vi "Get Profile Data.vi"(8 "error in (no error)":errorcluster, 10 "Bitfile Path":path, 11 "Profile Data In":T1[](array[typedef])) -> (1 "List of IO interfaces":T2[](array[typedef]), 3 "Profile Data Out":T1[](array[typedef]))   [LabVIEW 2021]
uses:
  <vilib>/myRIO/Common/Instrument Driver Framework/Utilities/typedefs/Hardware Version Enum.ctl
  <vilib>/myRIO/Common/Profile Manager Framework/typedefs/Channel Type Profile.ctl
  <vilib>/myRIO/Common/Instrument Driver Framework/Utilities/typedefs/Channel Types.ctl
  <vilib>/myRIO/Common/Profile Manager Framework/typedefs/Channel Info.ctl
  <vilib>/myRIO/Common/Instrument Driver Framework/Utilities/typedefs/Channel List Array.ctl
  <vilib>/myRIO/Common/Instrument Driver Framework/Utilities/typedefs/Channel List Cluster.ctl
  <vilib>/rvi/Bitfile/niFpgaBitfileReadAction.ctl
panel:
  out "Read Bitfile Time":u32
  in  "Hardware Version":T4=enum."myRIO-1900"
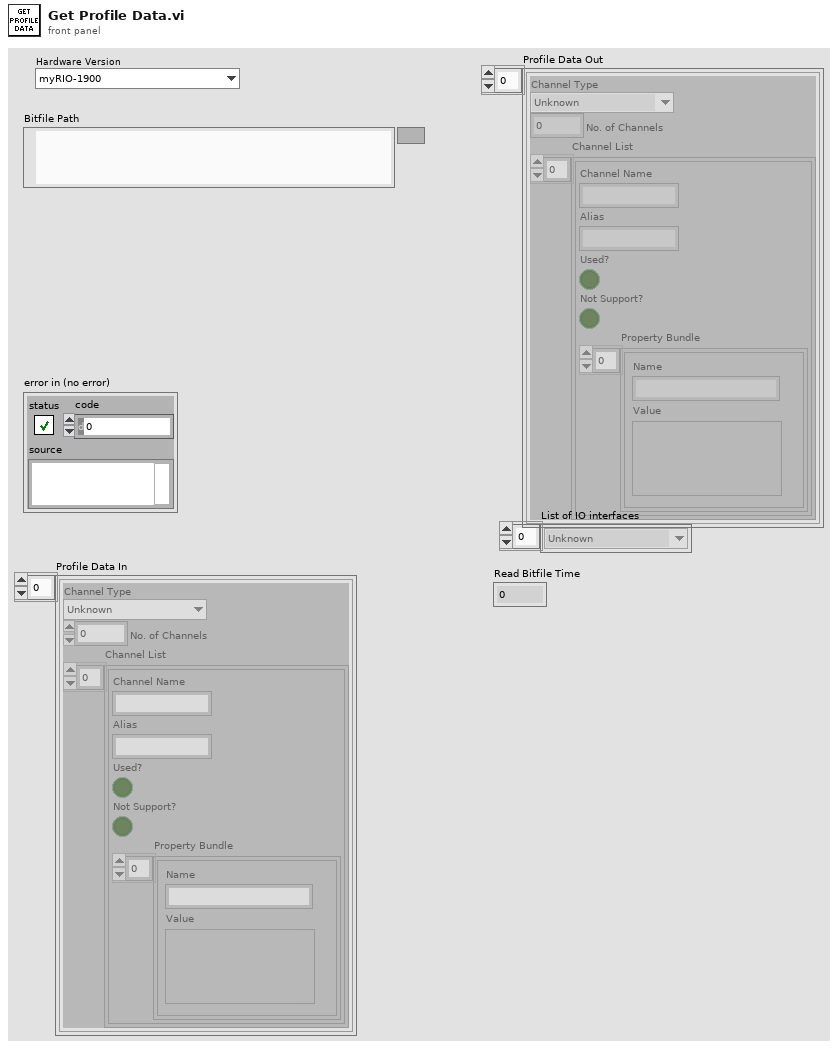
[diagram p1: front panel]
types:
  T1 = typedef "Channel Type Profile.ctl" = cluster{"Channel Type":T2, "No. of Channels":dbl, "Channel List":T3[]}
  T2 = typedef "Channel Types.ctl" = enum32{"Unknown", "AI", "AO", "DIO - DI", "DIO", "DIO - DO", "I2C", "PWM", "Encoder", "SPI", "UART", "Accelerometer", "DIO - LED", "DIO - Button", "AI (N Samples)", "AudioIn (N Samples)", "AO (N Samples)", "AudioOut (N Samples)", "DI (N Samples)", "DO (N Samples)", "AI IRQ", "DI IRQ", "Timer IRQ", "RSL", "Relay", "CAN", "AI (Continuous)", "AO (Continuous)"}
  T3 = typedef "Channel Info.ctl" = cluster{"Channel Name":string, "Alias":string, "Used?":bool, "Not Support?":bool, "Property Bundle":cluster{"Name":string, "Value":variant}[]}
  T4 = typedef "Hardware Version Enum.ctl" = enum16{"Unknown", "myRIO-1900", "myRIO-1950", "roboRIO", "NI ELVIS RIO CM", "ELVIS III"}
  T5 = typedef "niFpgaBitfileReadAction.ctl" = enum16{"<all>", "BitfileInfo", "ViInfo", "ProjectInfo"}
  T6 = typedef "niFpgaBitfileStructure.ctl" = cluster{"Bitfile":T7, "VI":T8, "Project":T15}
  T7 = typedef "niFpgaBitfileStructure_Bitfile.ctl" = cluster{"SignatureRegister":u8[], "SignatureGuids":u8[], "SignatureNames":u8[], "SignatureBitstream":u8[], "TimeStamp":string, "CompileStatus":string, "BitstreamVersion":u32}
  T8 = typedef "niFpgaBitfileStructure_VI.ctl" = cluster{"Name":string, "RegisterMap":T9[], "Icon":T14}
  T9 = typedef "nirviControlStructure.ctl" = cluster{"Name":string, "Hidden":bool, "Indicator":bool, "Flattened Type":string, "Grouping":cluster{"Grouped":bool, "Member Names":string[], "Member IDs":u32[]}, "Address":u32, "Size":u32, "Class":u32, "Internal":bool, "Typedef":T10, "ID":u32, "Bidirectional":bool, "Synchronous":bool, "Mechanical Action":T11, "Sub Controls":T12[], "Access May Timeout":bool, "Register Node":bool}
  T10 = typedef "nirviTypdefDescription.ctl" = cluster{"Typedef":bool, "Path":path}
  T11 = typedef "nirviMechanicalAction.ctl" = enum8{"Switch When Pressed", "Switch When Released", "Switch Until Released", "Latch When Pressed", "Latch When Released", "Latch Until Released"}
  T12 = typedef "nirviSubControlStructure.ctl" = cluster{"Name":string, "flattened Type":string, "Cluster Information":T13, "Typedef":T10}
  T13 = typedef "nirviClusterElementControl.ctl" = cluster{"Name Hierarchy":string[], "Item Order":u32[]}
  T14 = typedef "imagedata.ctl" = cluster{"image type":i32, "image depth":i32, "image":u8[], "mask":u8[], "colors":u32[], "Rectangle":cluster{"left":i16, "top":i16, "right":i16, "bottom":i16}}
  T15 = typedef "niFpgaBitfileStructure_Project.ctl" = cluster{"TargetClass":string, "AutoRunWhenDownloaded":bool, "CompilationResults":string, "MultipleUserClocks":bool, "AllowEnableRemoval":bool}
  T16 = typedef "Channel List Array.ctl" = T17[]
  T17 = typedef "Channel List Cluster.ctl" = cluster{"Channel List":string[]}
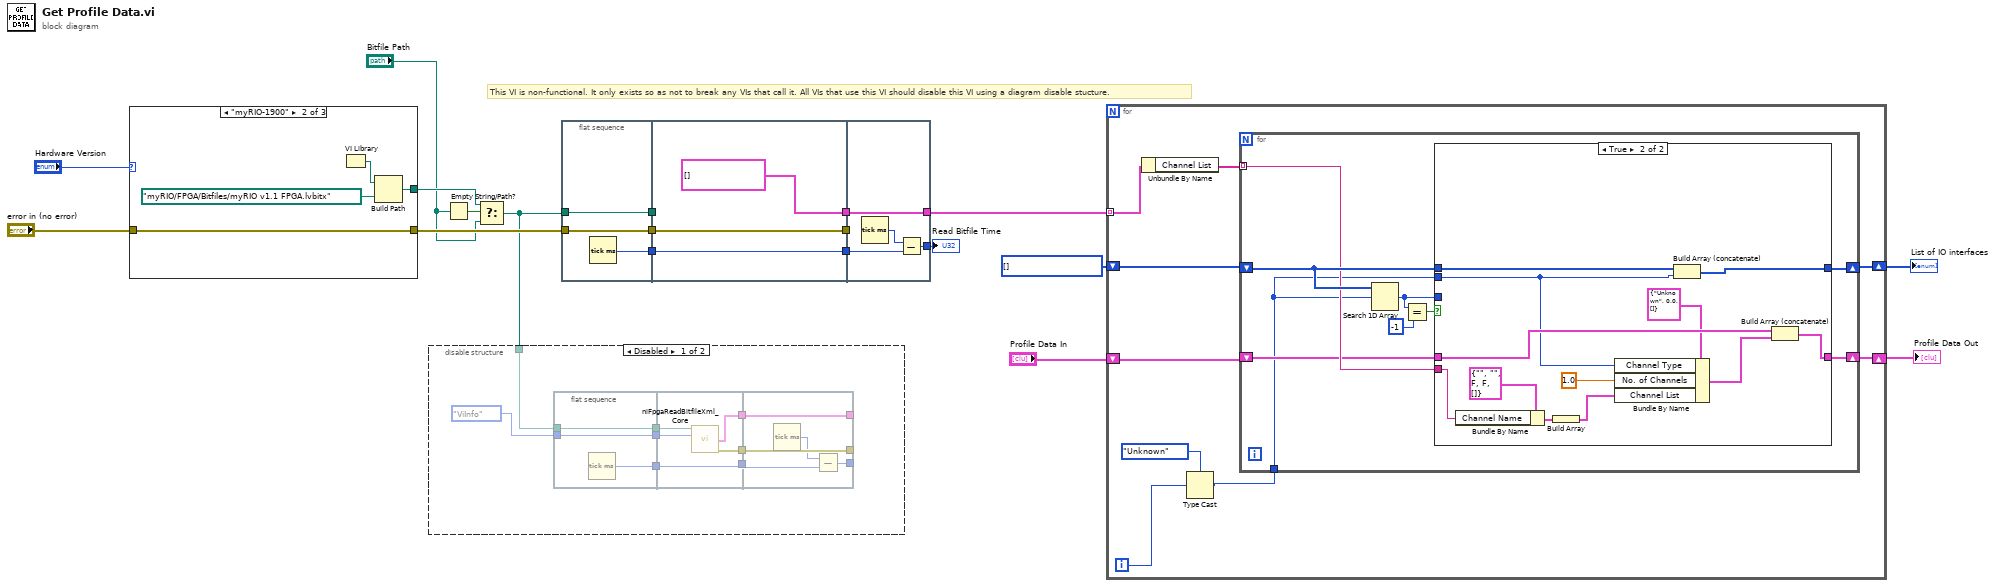
[diagram p0: block diagram]
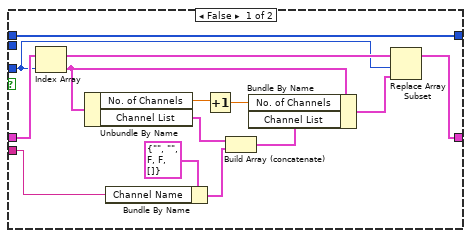
[diagram p2: hidden frame]
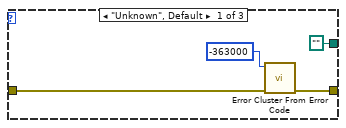
[diagram p4: hidden frame]
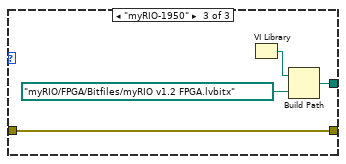
[diagram p5: hidden frame]
diagram:
  w2 = T2[] [] items=["Unknown", "AI", "AO", "DIO - DI", "DIO", "DIO - DO", "I2C", "PWM", "Encoder", "SPI", "UART", "Accelerometer", "DIO - LED", "DIO - Button", "AI (N Samples)", "AudioIn (N Samples)", "AO (N Samples)", "AudioOut (N Samples)", "DI (N Samples)", "DO (N Samples)", "AI IRQ", "DI IRQ", "Timer IRQ", "RSL", "Relay", "CAN", "AI (Continuous)", "AO (Continuous)"]
  # "This VI is non-functional. It only exists so as not to break any VIs that call it. All VIs that use this VI should disable this VI using a diagram disable stucture."
  n1 = case shown="\"myRIO-1900\"" "Hardware Version" {
    tunnel: [path "" w24 w28] -> w8
    tunnel: [w21 w25 w29] -> w18
    tunnel: "error in (no error)" -> [w20 w25 w29]
    frame "Unknown", Default {
      n2 = call <vilib>:"Error Cluster From Error Code.vi"("error in (no error)"=w20, "error code (0)"=-363000) -> ("error out"=w21:errorcluster)  [unwired: 7 in]
    }
    frame "myRIO-1900" {
      n3 = VI Library() -> (path=w27:path)
      n4 = Build Path(base path=w27, name or relative path=path "myRIO/FPGA/Bitfiles/myRIO v1.1 FPGA.lvbitx" ("bitfile path")) -> (appended path=w24:path)
    }
    frame "myRIO-1950" {
      n5 = VI Library() -> (path=w31:path)
      n6 = Build Path(base path=w31, name or relative path=path "myRIO/FPGA/Bitfiles/myRIO v1.2 FPGA.lvbitx" ("bitfile path")) -> (appended path=w28:path)
    }
  }
  n7 = Empty String/Path?(string/path="Bitfile Path") -> (empty?=w9:bool)
  n8 = Select(t=w8, s=w9, f="Bitfile Path") -> (s? t:f=w7:path)
  n9 = disable-structure shown="Disabled" {
    disable-tunnel: w7 -> [w32 _]
    frame Disabled {
      n10 = flat-sequence {
        tunnel: w32 -> [w41]
        tunnel: niFpgaBitfileReadAction."ViInfo" ("action") -> [w42]
        tunnel: [w42] -> w39
        tunnel: [w41] -> w38
        tunnel: [w40] -> w37
        tunnel: [w47] -> w36
        tunnel: [w45] -> w35
        tunnel: w39 -> [w46]
        tunnel: w38 -> [w44]
        tunnel: [w43] -> w34
        tunnel: w37 -> [w43]
        tunnel: [w51] -> _
        tunnel: [w52] -> _
        tunnel: w36 -> [w52]
        tunnel: w35 -> [w51]
        tunnel: w34 -> [w49]
        tunnel: [w48] -> _
        frame #0 {
          n11 = Tick Count (ms)() -> (millisecond timer value=w40:u32)
        }
        frame #1 {
          n12 = call <vilib>:"niFpgaReadBitfileXml_Core.vi"("bitfile path"=w44, "action"=w46) -> ("bitfile structure"=w47:T6, "error out"=w45:errorcluster)  [unwired: 2 in, 10 out]
        }
        frame #2 {
          n13 = Tick Count (ms)() -> (millisecond timer value=w50:u32)
          n14 = Subtract(x=w50, y=w49) -> (x-y=w48:u32)
        }
      }
    }
    frame Enabled {
    }
  }
  n15 = flat-sequence {
    tunnel: w7 -> [w54]
    tunnel: w18 -> [w55]
    tunnel: [w55] -> w15
    tunnel: [w54] -> w14
    tunnel: [w53] -> w11
    tunnel: w15 -> [w57]
    tunnel: w14 -> [_]
    tunnel: [T16 [] ("Channels Array")] -> w13
    tunnel: [w58] -> w12
    tunnel: w11 -> [w58]
    tunnel: [w57] -> w1
    tunnel: [w62] -> w4
    tunnel: w13 -> [w62]
    tunnel: w12 -> [w60]
    tunnel: [w59] -> w10
    tunnel: w1 -> [_]
    frame #0 {
      n16 = Tick Count (ms)() -> (millisecond timer value=w53:u32)
    }
    frame #1 {
    }
    frame #2 {
      n17 = Tick Count (ms)() -> (millisecond timer value=w61:u32)
      n18 = Subtract(x=w61, y=w60) -> (x-y=w59:u32)
    }
  }
  n19 = for {
    tunnel: w4 -> [w69] mode=indexing
    shift-right: [w71] -> w17
    shift-left: "Profile Data In" -> [w67]
    shift-right: [w70] -> w16
    shift-left: w2 -> [w66]
    i -> [w63]
    n20 = Unbundle By Name(w69) -> ("Channel List"=w68:string[])
    n21 = Type Cast(type=Channel_Types."Unknown" ("Channel Types"), x=w63) -> (*(type *) &x=w64:T2)
    n22 = for {
      tunnel: w68 -> [w76] mode=indexing
      shift-right: [w77] -> w70
      shift-left: w66 -> [w78]
      shift-right: [w74] -> w71
      shift-left: w67 -> [w75]
      tunnel: w64 -> [w72]
      n23 = Search 1D Array(1D array=w78, element=w72) -> (index of element=w73:i32)  [unwired: 1 in]
      n24 = Equal?(x=w73, y=-1) -> (x = y?=w79:bool)
      n25 = case shown="True" w79 {
        tunnel: w78 -> [w93 w105]
        tunnel: [w93 w104] -> w77
        tunnel: w72 -> [_ w102]
        tunnel: w76 -> [w86 w100]
        tunnel: w75 -> [w89 w103]
        tunnel: [w82 w96] -> w74
        tunnel: w73 -> [w88 _]
        frame False {
          n26 = Index Array(array=w89, index=w88) -> (element=w92:T1)
          n27 = Unbundle By Name(w92) -> ("No. of Channels"=w91:dbl, "Channel List"=w85:T3[])
          n28 = Bundle By Name(cluster=T3 {"Channel Name"="", "Alias"="", "Used?"=FALSE, "Not Support?"=FALSE, "Property Bundle"=[]} ("Channel Info"), "Channel Name"=w86) -> (w84:T3)
          n29 = Increment(x=w91) -> (x+1=w90:dbl)
          n30 = Build Array (concatenate)(w85, w84) -> (w83:T3[])
          n31 = Bundle By Name(cluster=w92, "No. of Channels"=w90, "Channel List"=w83) -> (w87:T1)
          n32 = Replace Array Subset(array=w89, new element=w87, index=w88) -> (w82:T1[])
        }
        frame True {
          n33 = Bundle By Name(cluster=T3 {"Channel Name"="", "Alias"="", "Used?"=FALSE, "Not Support?"=FALSE, "Property Bundle"=[]} ("Channel Info"), "Channel Name"=w100) -> (w99:T3)
          n34 = Build Array(w99) -> (w98:T3[])
          n35 = Bundle By Name(cluster=T1 {"Channel Type"=enum."Unknown", "No. of Channels"=0.0, "Channel List"=[]} ("Channel Type Profile Out"), "Channel Type"=w102, "No. of Channels"=1.0, "Channel List"=w98) -> (w97:T1)
          n36 = Build Array (concatenate)(w105, w102) -> (w104:T2[])
          n37 = Build Array (concatenate)(w103, w97) -> (w96:T1[])
        }
      }
    }
  }
  "Profile Data Out" <- w17
  "List of IO interfaces" <- w16
  "Read Bitfile Time" <- w10
